vi "NotInWordList.vi"(8 "error in (no error)":errorcluster) -> (0 "error out":errorcluster)   [LabVIEW 2024, in "GUI.lvlib" / "View.lvclass"]
uses:
  View.lvclass
panel:
  # "Not in word list"
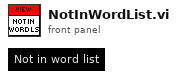
[diagram p1: front panel]
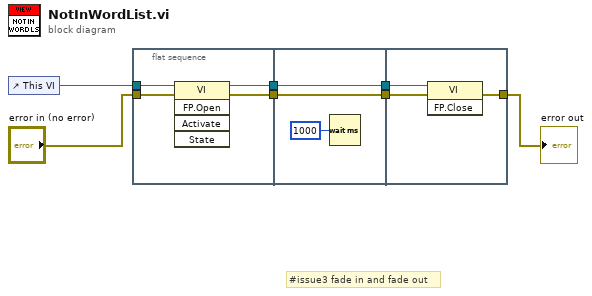
[diagram p0: block diagram]
diagram:
  # "#issue3 fade in and fade out"
  n1 = control-ref of="This VI"() -> (w7:refnum<vi>)
  n2 = flat-sequence {
    tunnel: w7 -> [w11]
    tunnel: "error in (no error)" -> [w10]
    tunnel: [w9] -> w5
    tunnel: [w8] -> w4
    tunnel: w5 -> [w13]
    tunnel: w4 -> [w12]
    tunnel: [w13] -> w3
    tunnel: [w12] -> w2
    tunnel: w3 -> [w17]
    tunnel: w2 -> [w16]
    tunnel: [w15] -> w1
    frame #0 {
      n3 = invoke class="VI" method="FP.Open"(reference=w11, error in=w10) -> (reference out=w9:refnum<vi>, error out=w8:errorcluster)  [unwired: 3 in, 3 out]
    }
    frame #1 {
      n4 = Wait (ms)(milliseconds to wait=u32 1000) -> ()  [unwired: 1 out]
    }
    frame #2 {
      n5 = invoke class="VI" method="FP.Close"(reference=w17, error in=w16) -> (error out=w15:errorcluster)  [unwired: 1 in, 2 out]
    }
  }
  "error out" <- w1
